vi "Pixy I2C.vi"() -> ()   [LabVIEW 2016]
doc: "This example shows how to communicate and interpret data for a PIXY camera."
uses:
  <vilib>/Rock Robotics/SystemInterfaces/i2clib/i2c_bus.ctl
  <vilib>/Rock Robotics/WPI/SPI/WPI_SPIMode.ctl
panel:
  in  "CC Objects":bool=TRUE
  in  "Objects":bool=TRUE
  out "CC Objects":T1(array[cluster])
  out "Totals":T2
  in  "I2C Bus":T3
  in  "Device Address":u8=84 format="%.0x"
  in  "Image Brightness":u8(slide)=80 scale=0.0..255.0
  out "ms between frames":u32(graph)
  in  "Shape Colors":u32[](array[colorbox])=[16748288, 16746709, 1244948]
  in  "LED Color":cluster{"Red":u8, "Green":u8, "Blue":u8} {"Blue" scale=0.0..255.0; "Green" scale=0.0..255.0; "Red" scale=0.0..255.0}
  out "Picture":picture
  out "Objects":T4(array[cluster])
  # "Top left of roboRIO"
  # "Back of PIXY"
  # "1  2\n 3  4\n 5  6\n 7  8\n 9 10"
  # "I2C cable\nPIXY      roboRIO\nPin 5 ----- SCL\nPin 9 ----- SDA\nPin 10 --- GND"
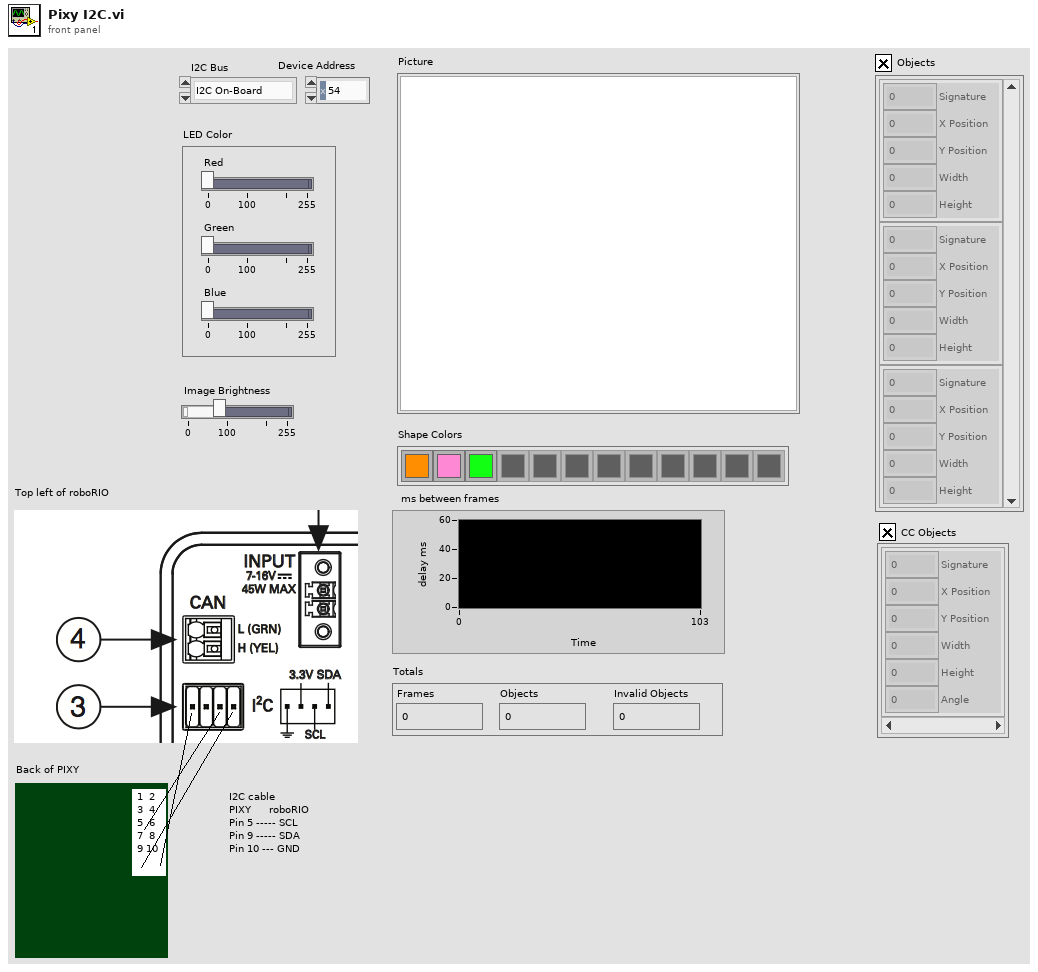
[diagram p1: front panel]
types:
  T1 = cluster{"Signature":u16, "X Position":u16, "Y Position":u16, "Width":u16, "Height":u16, "Angle":i16}[]
  T2 = cluster{"Frames":u32, "Objects":u32, "Invalid Objects":i32}
  T3 = typedef "i2c_bus.ctl" = enum16{"I2C On-Board", "I2C MXP", "Invalid"}
  T4 = cluster{"Signature":u16, "X Position":u16, "Y Position":u16, "Width":u16, "Height":u16}[]
  T5 = enum16{"Read Objects", "Write LED Color", "Write Brightness", "Write Objects", "Read Settings"}
  T6 = typedef "WPI_SPIMode.ctl" = enum16{"Mode 0 (Clk Idle Low,Sample on Leading)", "Mode 1 (Clk Idle Low,Sample on Trailing)", "Mode 2 (Clk Idle High,Sample on Leading)", "Mode 3 (Clk Idle High,Sample on Trailing)"}
  T7 = typedef "WPI_SPIDevRef.ctl" = cluster{"DevStatus":errorcluster, "Handle":i32, "SPI Bus":T8}
  T8 = typedef "spi_bus.ctl" = enum16{"SPI On-Board, CS0", "SPI On-Board, CS1", "SPI On-Board, CS2", "SPI On-Board, CS3", "SPI MXP", "Invalid"}
  T9 = typedef "WPI_I2CDevRef.ctl" = cluster{"DevStatus":errorcluster, "Device Address":u8, "Handle":i32, "I2C Bus":T3}
  T10 = cluster{"Signature":u16, "X Position":u16, "Y Position":u16, "Width":u16, "Height":u16}
  T11 = cluster{"Signature":u16, "X Position":u16, "Y Position":u16, "Width":u16, "Height":u16, "Angle":i16}
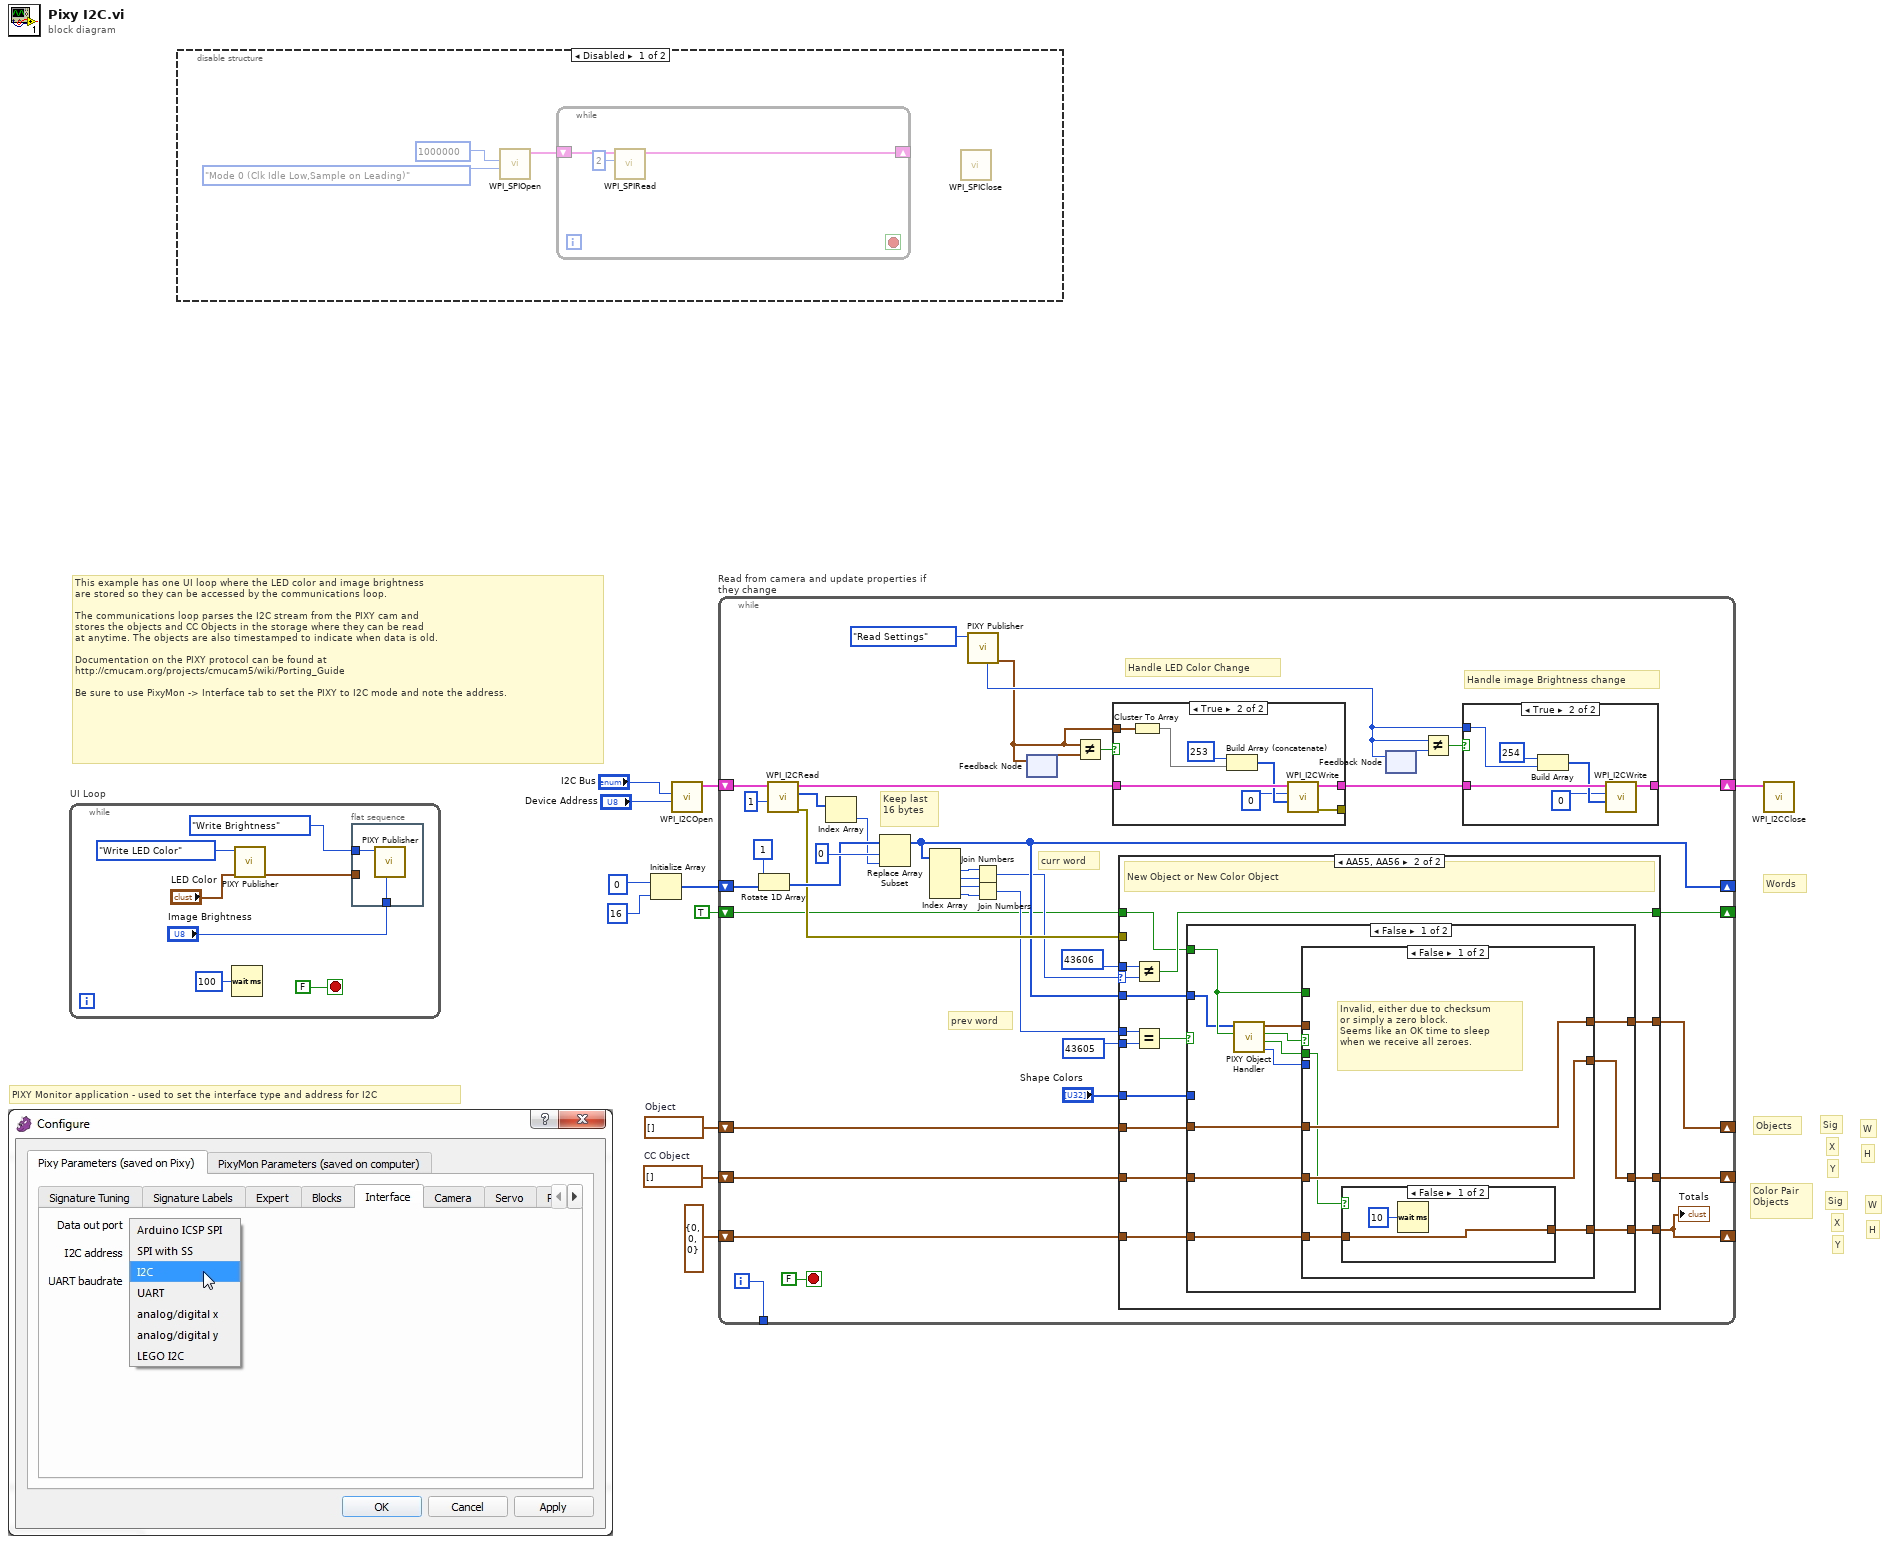
[diagram p0: block diagram]
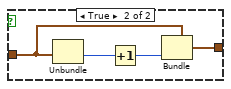
[diagram p3: hidden frame]
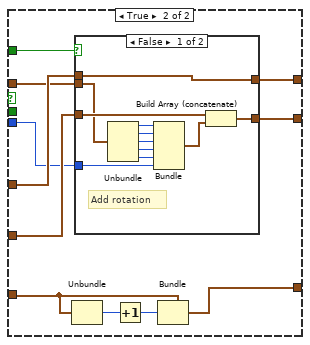
[diagram p4: hidden frame]
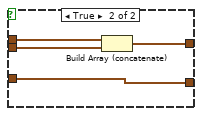
[diagram p5: hidden frame]
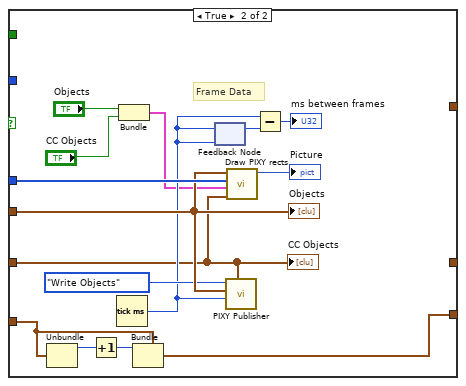
[diagram p6: hidden frame]
diagram:
  w4 = T1 []  # CC Object
  w5 = T4 []  # Object
  # "PIXY Monitor application - used to set the interface type and address for I2C"
  # "This example has one UI loop where the LED color and image brightness\nare stored so they can be accessed by the communications loop.\n\nThe communications loop parses the I2C stream from the PIXY cam and\nstores the objects and CC Objects in the storage where they can be read\nat anytime. The objects are also timestamped to indicate when data is old.\n\nDocumentation on the PIXY protocol can be found at\nhttp://cmucam.org/projects/cmucam5/wiki/Porting_Guide\n\nBe sure to use PixyMon -> Interface tab to set the PIXY to I2C mode and note the address."
  # "H"
  # "W"
  # "Y"
  # "X"
  # "Sig"
  # "Color Pair\nObjects"
  # "H"
  # "W"
  # "Y"
  # "X"
  # "Sig"
  # "Objects"
  # "Words"
  n1 = while "UI Loop" {
    stop <- FALSE stop-if-true
    n2 = Wait (ms)(milliseconds to wait=u32 100) -> ()  [unwired: 1 out]
    n3 = call "PIXY Publisher.vi"("Color"="LED Color", "Operation"=T5."Write LED Color") -> ("Color Out"=w13:cluster{"Red":u8, "Green":u8, "Blue":u8})  [unwired: 5 in, 4 out]
    n4 = flat-sequence {
      tunnel: T5."Write Brightness" ("Operation") -> [w20]
      tunnel: "Image Brightness" -> [w19]
      tunnel: w13 -> [_]
      frame #0 {
        n5 = call "PIXY Publisher.vi"("Brightness"=w19, "Operation"=w20) -> ()  [unwired: 5 in, 5 out]
      }
    }
  }
  n6 = disable-structure shown="Disabled" {
    frame Disabled {
      n7 = call <vilib>:"WPI_SPIOpen.vi"("Mode (3)"=WPI_SPIMode."Mode 0 (Clk Idle Low,Sample on Leading)", "Clock Rate (Hz)"=1000000) -> ("SPIDevRef"=w21:T7)  [unwired: 4 in, 5 out]
      n8 = while {
        shift-right: [w24] -> _
        shift-left: w21 -> [w26]
        stop <- _ stop-if-true
        n9 = call <vilib>:"WPI_SPIRead.vi"("Num to Read"=2, "SPIDevRef"=w26) -> ("SPIDevRef"=w24:T7)  [unwired: 7 in, 2 out]
      }
      n10 = call <vilib>:"WPI_SPIClose.vi"() -> ()  [unwired: 11 in, 1 out]
    }
    frame Enabled {
    }
  }
  n11 = Initialize Array(u8 0 ("Num to Read"), 16 ("Num to Read")) -> (w6:u8[])
  n12 = call <vilib>:"WPI_I2COpen.vi"("Device Address"="Device Address", "I2C Bus"="I2C Bus") -> ("I2CDevRef"=w3:T9)  [unwired: 2 in, 7 out]
  n13 = while "Read from camera and update properties if they change" {
    shift-right: [w51] -> w9
    shift-left: w3 -> [w65]
    shift-right: [w33] -> _
    shift-left: w6 -> [w56]
    shift-right: [w59] -> _
    shift-left: w5 -> [w60]
    tunnel: [w58] -> _
    shift-right: [w49] -> _
    shift-left: w4 -> [w50]
    shift-right: [w29] -> _
    shift-left: T2 {"Frames"=0, "Objects"=0, "Invalid Objects"=0} ("Totals") -> [w30]
    shift-right: [w27] -> _
    shift-left: TRUE -> [w28]
    i -> [w58]
    stop <- FALSE stop-if-true
    # "curr word"
    # "Handle image Brightness change"
    # "Handle LED Color Change"
    # "prev word"
    # "Keep last\n16 bytes"
    n14 = Rotate 1D Array(1:w56, 2:1 ("Num to Read")) -> (0:w57:u8[])
    n15 = call <vilib>:"WPI_I2CRead.vi"("I2CBytesToRead"=u8 1, "I2CDevRef"=w65) -> ("error out"=w40:errorcluster, "Data Out"=w63:u8[], "I2CDevRef"=w55:T9)  [unwired: 7 in]
    n16 = Index Array(array=w63) -> (element=w39:u8)  [unwired: 1 in]
    n17 = Replace Array Subset(array=w57, new element=w39, index=0 ("Num to Read")) -> (w33:u8[])
    n18 = Index Array(array=w33) -> (element #1=w38:u8, element #2=w37:u8, element #3=w36:u8, element #4=w35:u8)  [unwired: 4 in]
    n19 = call "PIXY Publisher.vi"("Operation"=T5."Read Settings") -> ("Color Out"=w46:cluster{"Red":u8, "Green":u8, "Blue":u8}, "Brightness Out"=w47:u8)  [unwired: 6 in, 3 out]
    n20 = Join Numbers(hi=w38, lo=w37) -> ((hi.lo)=w32:u16)
    n21 = Join Numbers(hi=w36, lo=w35) -> ((hi.lo)=w34:u16)
    n22 = feedback #1() -> (w54:cluster{"Red":u8, "Green":u8, "Blue":u8})  [unwired: 1 in]
    n23 = feedback-in #1(w46) -> ()
    n24 = Not Equal?(x=w46, y=w54) -> (x != y?=w53:bool)
    n25 = case shown="True" w53 {
      tunnel: w55 -> [w156 w164]
      tunnel: [w156 w163] -> w52
      tunnel: w46 -> [_ w162]
      tunnel: [_ w158] -> _
      frame False {
      }
      frame True {
        n26 = Cluster To Array(cluster=w162) -> (array=w161:u8[])
        n27 = Build Array (concatenate)(u8 253 ("Num to Read"), w161) -> (w160:u8[])
        n28 = call <vilib>:"WPI_I2CWrite.vi"("I2CDataToSend"=w160, "I2CRegister"=0 ("Num to Read"), "I2CDevRef"=w164) -> ("error out"=w158:errorcluster, "I2CDevRef"=w163:T9)  [unwired: 7 in]
      }
    }
    n29 = case shown="AA55, AA56" w32 {
      selector: w32 -> [_ w79]
      tunnel: w34 -> [_ w84]
      tunnel: u16 43605 ("Num to Read") -> [_ w83]
      tunnel: w60 -> [w69 w82]
      tunnel: [w69 w81] -> w59
      tunnel: w33 -> [_ w75]
      tunnel: u16 43606 ("Num to Read") -> [_ w78]
      tunnel: w50 -> [w68 w77]
      tunnel: [w68 w76] -> w49
      tunnel: w40 -> [_ _]
      tunnel: "Shape Colors" -> [_ w74]
      tunnel: w30 -> [w67 w73]
      tunnel: [w67 w72] -> w29
      tunnel: w28 -> [w66 w70]
      tunnel: [w66 w71] -> w27
      frame Default {
        # "Nothing to do, already appended"
        # "Just another word for the object"
      }
      frame 43605, 43606 {
        # "New Object or New Color Object"
        n30 = Not Equal?(x=w78, y=w79) -> (x != y?=w71:bool)
        n31 = Equal?(x=w84, y=w83) -> (x = y?=w80:bool)
        n32 = case shown="False" w80 {
          tunnel: w82 -> [w96 w144]
          tunnel: [w95 _] -> w81
          tunnel: w74 -> [_ w146]
          tunnel: w77 -> [w94 w137]
          tunnel: w70 -> [w89 _]
          tunnel: [w93 _] -> w76
          tunnel: w75 -> [w87 _]
          tunnel: w73 -> [w86 w141]
          tunnel: [w85 w140] -> w72
          frame False {
            n33 = call "PIXY Object Handler.vi"("Normal Object"=w89, "Accumulated Words"=w87) -> ("Angle"=w88:i16, "CheckSum Error"=w90:bool, "Valid"=w91:bool, "Object"=w92:T10)  [unwired: 6 in]
            n34 = case shown="False" w91 {
              tunnel: w96 -> [w101 w118]
              tunnel: [w101 w117] -> w95
              tunnel: w94 -> [w100 w116]
              tunnel: w89 -> [_ w115]
              tunnel: [w100 w114] -> w93
              tunnel: w92 -> [_ w113]
              tunnel: w90 -> [w99 _]
              tunnel: w88 -> [_ w112]
              tunnel: w86 -> [w98 w111]
              tunnel: [w97 w110] -> w85
              frame False {
                # "Invalid, either due to checksum\nor simply a zero block.\nSeems like an OK time to sleep\nwhen we receive all zeroes."
                n35 = case shown="False" w99 {
                  tunnel: w98 -> [w103 w105]
                  tunnel: [w103 w107] -> w97
                  frame False {
                    n36 = Wait (ms)(milliseconds to wait=u32 10) -> ()  [unwired: 1 out]
                  }
                  frame True {
                    n37 = Unbundle(w105) -> ("Invalid Objects"=w106:i32)  [unwired: 2 out]
                    n38 = Increment(x=w106) -> (x+1=w104:i32)
                    n39 = Bundle(cluster=w105, "Invalid Objects"=w104) -> (w107:T2)  [unwired: 2 in]
                  }
                }
              }
              frame True {
                n40 = Unbundle(w111) -> ("Objects"=w109:u32)  [unwired: 2 out]
                n41 = case shown="False" w115 {
                  tunnel: w113 -> [w123 w133]
                  tunnel: w118 -> [w129 w132]
                  tunnel: [w129 w131] -> w117
                  tunnel: w116 -> [w128 w130]
                  tunnel: [w127 w130] -> w114
                  tunnel: w112 -> [w119 _]
                  frame False {
                    # "Add rotation"
                    n42 = Unbundle(w123) -> ("Signature"=w125:u16, "X Position"=w124:u16, "Y Position"=w122:u16, "Width"=w121:u16, "Height"=w120:u16)
                    n43 = Bundle("Signature"=w125, "X Position"=w124, "Y Position"=w122, "Width"=w121, "Height"=w120, "Angle"=w119) -> (w126:T11)  [unwired: 1 in]
                    n44 = Build Array (concatenate)(w128, w126) -> (w127:T1)
                  }
                  frame True {
                    n45 = Build Array (concatenate)(w132, w133) -> (w131:T4)
                  }
                }
                n46 = Increment(x=w109) -> (x+1=w108:u32)
                n47 = Bundle(cluster=w111, "Objects"=w108) -> (w110:T2)  [unwired: 2 in]
              }
            }
          }
          frame True {
            # "Frame Data"
            n48 = Unbundle(w141) -> ("Frames"=w139:u32)  [unwired: 2 out]
            n49 = Increment(x=w139) -> (x+1=w138:u32)
            n50 = Tick Count (ms)() -> (millisecond timer value=w142:u32)
            n51 = Bundle("Objects"="Objects", "CC Objects"="CC Objects") -> (w136:cluster{"Objects":bool, "CC Objects":bool})  [unwired: 1 in]
            n52 = Bundle(cluster=w141, "Frames"=w138) -> (w140:T2)  [unwired: 2 in]
            n53 = feedback #2(w142) -> (w148:u32)
            n54 = feedback-in #2(w142) -> ()
            n55 = call "PIXY Publisher.vi"("Color Combo Object"=w137, "TimeStamp in"=w142, "Object"=w144, "Operation"=T5."Write Objects") -> ()  [unwired: 3 in, 5 out]
            n56 = call "Draw PIXY rects.vi"("CC Objects"=w137, "Draw Options"=w136, "Colors"=w146, "Object"=w144) -> ("Picture"=→"Picture":picture)  [unwired: 7 in]
            n57 = Subtract(x=w142, y=w148) -> (x-y=→"ms between frames":u32)
            "Objects" <- w144
            "CC Objects" <- w137
          }
        }
      }
    }
    "Totals" <- w29
    n58 = feedback #3() -> (w45:u8)  [unwired: 1 in]
    n59 = feedback-in #3(w47) -> ()
    n60 = Not Equal?(x=w47, y=w45) -> (x != y?=w44:bool)
    n61 = case shown="True" w44 {
      tunnel: w52 -> [w149 w155]
      tunnel: [w149 w154] -> w51
      tunnel: w47 -> [_ w150]
      frame False {
      }
      frame True {
        n62 = Build Array(u8 254 ("Num to Read"), w150) -> (w152:u8[])
        n63 = call <vilib>:"WPI_I2CWrite.vi"("I2CDataToSend"=w152, "I2CRegister"=0 ("Num to Read"), "I2CDevRef"=w155) -> ("I2CDevRef"=w154:T9)  [unwired: 7 in, 1 out]
      }
    }
  }
  n64 = call <vilib>:"WPI_I2CClose.vi"("I2CDevRef"=w9) -> ()  [unwired: 10 in, 1 out]
